vi "ROI entry-Event handler-Completion.vi"(7 "Adj Timing for MC":bool, 11 "Ctrl ref of the control that caused the user event":refnum<vi>) -> (1 "Exit":bool=TRUE, 3 "Imaging Mode":T1)   [LabVIEW 2020]
uses:
  Typedefs/Top level VI states.ctl
  Typedefs/Save-Load enum.ctl
  Typedefs/Which path.ctl
  Visualisation/Functional Imaging Viewer/SubVIs/Experiment header interface/Typedefs/Header file interface module functions enum.ctl
  Visualisation/Functional Imaging Viewer/SubVIs/Experiment header interface/Typedefs/Header file sections.ctl
  Visualisation/Functional Imaging Viewer/SubVIs/Experiment header interface/Typedefs/Header file type enum.ctl
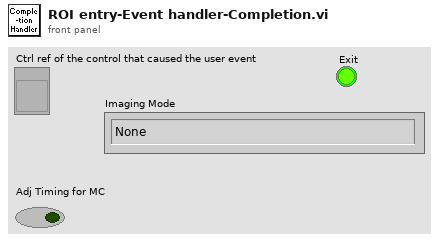
[diagram p1: front panel]
types:
  T1 = typedef "Top level VI states.ctl" = enum16{"None", "Initialise UI", "<STACK PROTOCOL STATES>", "AOL Zstack-START", "AOL Zstack-STOP", "Motor Zstack-START", "Motor Zstack-STOP", "<ACQUISITION PROTOCOL STATES> ", "Functional Acquisition-START", "Functional Acquisition-STOP", "Single Plane Acquisition-START", "Single Plane Acquisition-STOP", "Volume Acquisition-START", "Volume Acquisition-STOP", "<LIVE IMAGING PROTOCOL STATES>", "Live Imaging-START", "Live Imaging-STOP", "Live Plane Imaging-START", "Live Plane Imaging-STOP", "Live Volume Imaging-START", "Live Volume Imaging-STOP", "<MOVEMENT CORRECTION PROTOCOL STATES>", "EXIT"}
  T2 = typedef "Which path.ctl" = enum16{"Configuration Files", "Calibration Files", "Images", "Setup.ini", "Loaded User profile.ini", "User's-Previous session.ini", "New user profile.ini", "Selected User profile.ini", "User profiles folder", "Power meter scaling.txt", "FOV Cal.ini", "Calibration.ini"}
  T3 = typedef "Save-Load enum.ctl" = enum16{"Save to file", "Load from file", "Compare from file", "Save Backup"}
  T4 = typedef "Header file sections.ctl" = enum16{"ALL SECTIONS", "LOGIN", "GLOBAL PARAMETERS", "CALIBRATION DATA", "IMAGING MODES", "TIME SERIES", "MOTOR Z-STACK", "AOL Z-STACK", "FUNCTIONAL IMAGING", "VOLUME IMAGING", "MOVEMENT CORRECTION", "CALIBRATION", "STATISTICS", "BIOLOGY INFORMATION"}
  T5 = typedef "Header file interface module functions enum.ctl" = enum16{"Load experiment header file", "Save experiment header file", "Clear stored values", "Read stored values", "Update specific value in memory", "Update values in memory"}
  T6 = typedef "Header file type enum.ctl" = enum16{"All parameters", "Params for funct acq w ROI or mscn", "Params for funct acq w rectangles", "Live imaging header parameters", "AOL Parameters"}
  T7 = typedef "ROI parameters data type.ctl" = cluster{"ROI index":dbl, "ROI ID":dbl, "ROI Time (ns)":dbl, "Pixels in ROI":dbl, "X start":dbl, "Y start":dbl, "Z start":dbl, "X stop":dbl, "Y stop":dbl, "Z stop":dbl, "Angle (deg)":dbl, "Composite ID":dbl, "Number of lines":dbl, "Frame Size":dbl, "Zoom":dbl, "Laser Power (%)":dbl, "ROI group ID":dbl, "Resolution":dbl, "Dwell Time per pixel":dbl, "Pixels per miniscan":dbl, "Original FOV (um)":dbl, "Apparent Frame Size":dbl, "Z Plane Idx":i32[], "Z Plane codes":i32[]}
  T8 = typedef "AOL_Globals.ctl" = cluster{"Imaging Protocol":T9, "Number of POI":u16, "Number of Miniscans":u16, "Number of Trials":u16, "Number of Cycles ":u64, "# Averaged Frames":u16, "Laser power (%)":u8, "Pockels (V)":dbl, "Acquisition Length (sec)":dbl, "Fill time (us)":dbl, "POI Dwell time (us)":dbl, "Miniscan Dwell time per pixel (us)":dbl, "PMT 1":dbl, "PMT 2":dbl, "Back Apperture (mA)":dbl, "Frame Size":T10, "Center Frequency":dbl, "Field of View (norm)":dbl, "DwellTime (us)":dbl, "Wavelength (nm)":dbl, "Zoom":dbl, "AOL Z":dbl, "AOL Mode":T11, "GridXY":dbl, "GridZ":dbl, "TriggerPeriod (sec)":dbl, "Number of Pixels in Miniscan":u16, "Experiment folder path":path, "X centre":dbl, "Y centre":dbl, "Angle (degrees)":dbl, "Plane Mode":T12, "Threshold":u16[], "Regenerate Chirps":bool, "Rectangle ROI length (pixels)":u16, "Rectangle ROI height (pixels)":u16, "AOD fill":u16, "StartupDelay":i32, "Samples Wait after Trigger":u16, "Slip Cycle":u32, "Add Cycle":bool, "Functional Mode":T13, "Z Start":dbl, "Z Stop":dbl, "# Planes":i32, "Total Pixels":i32, "Variable Miniscan Pixels":u16[], "Use Variable Length":bool, "Use Variable Resolution":bool, "Laser power (%) at Z Start":u8, "Laser power (%) at Z Stop":u8, "Ref Z Step":i8, "Ref Dwell Time (us)":dbl, "Field of View (um)":dbl}
  T9 = typedef "Imaging Protocols enum.ctl" = enum16{"AOL Z-Stack", "Motor Z Stack", "Functional Acquisition", "Single Plane Acquisition", "Volume Acquisition", "Live Imaging", "Live Plane Imaging", "Live Volume Imaging"}
  T10 = typedef "Frame Size.ctl" = u16
  T11 = typedef "AOL modes.ctl" = enum16{"Raster", "Structural", "Pointing", "Mini Scan", "Alignment"}
  T12 = typedef "Plane Mode.ctl" = u16
  T13 = typedef "Functional Mode.ctl" = enum16{"Point", "Line", "Patch", "Plane", "Volume"}
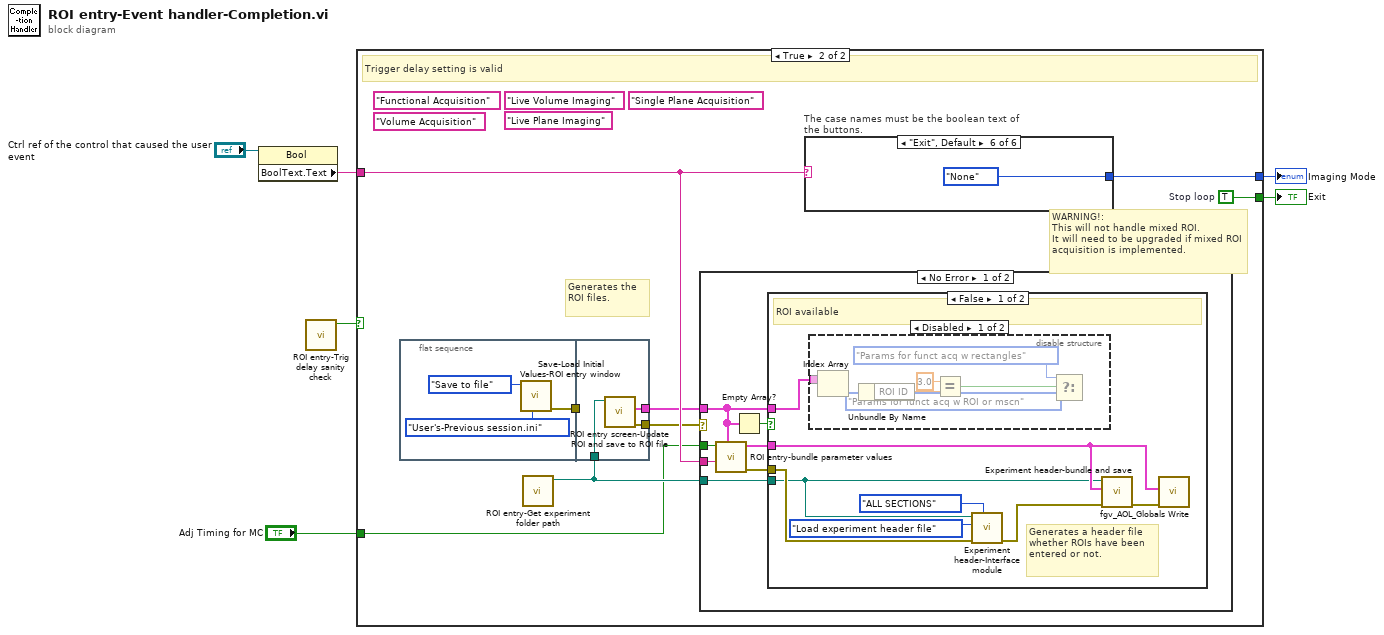
[diagram p0: block diagram]
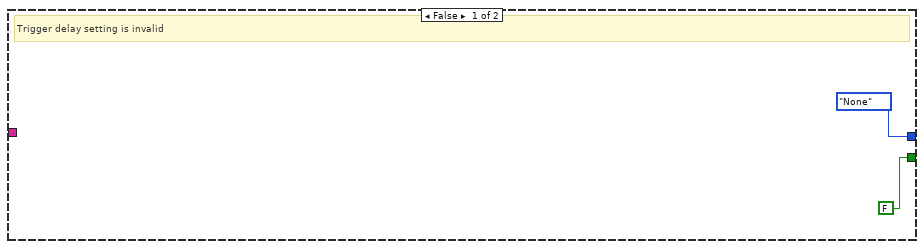
[diagram p2: hidden frame]
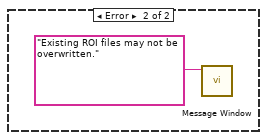
[diagram p5: hidden frame]
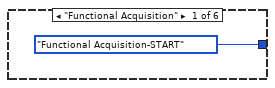
[diagram p6: hidden frame]
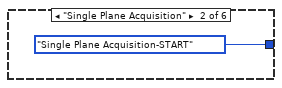
[diagram p7: hidden frame]
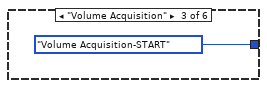
[diagram p8: hidden frame]
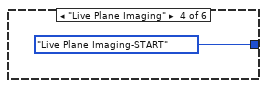
[diagram p9: hidden frame]
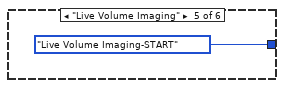
[diagram p10: hidden frame]
diagram:
  n1 = property on="Property Node" class="Bool"(reference="Ctrl ref of the control that caused the user event") -> ("BoolText.Text"=w6:string)  [unwired: 1 in, 2 out]
  n2 = call "ROI entry-Trig delay sanity check.vi"() -> ("Trigger delay is valid"=w2:bool)  [unwired: 10 in, 1 out]
  n3 = case shown="True" w2 {
    tunnel: w6 -> [_ w15]
    tunnel: [Top_level_VI_states."None" ("Imaging Mode") w12] -> w5
    tunnel: [FALSE ("Stop loop") w11] -> w3
    tunnel: "Adj Timing for MC" -> [_ w9]
    frame False {
      # "Trigger delay setting is invalid"
    }
    frame True {
      w11 = TRUE  # Stop loop
      (unwired) "Live Plane Imaging" ("Boolean Text.Text")
      (unwired) "Single Plane Acquisition" ("Boolean Text.Text")
      (unwired) "Live Volume Imaging" ("Boolean Text.Text")
      (unwired) "Functional Acquisition" ("Boolean Text.Text")
      (unwired) "Volume Acquisition" ("Boolean Text.Text")
      # "WARNING!:\nThis will not handle mixed ROI.\nIt will need to be upgraded if mixed ROI acquisition is implemented."
      # "Generates the ROI files."
      # "Trigger delay setting is valid"
      n4 = flat-sequence {
        tunnel: [w17] -> w10
        tunnel: w16 -> [w22]
        tunnel: [w21] -> w14
        tunnel: [w20] -> w13
        tunnel: w10 -> [_]
        frame #0 {
          n5 = call "Save-Load Initial Values-ROI entry window.vi"("Which file? (User profile.ini)"=Which_path."User's-Previous session.ini", "Function"=Save-Load_enum."Save to file") -> ("error out"=w17:errorcluster)  [unwired: 9 in]
        }
        frame #1 {
          n6 = call "ROI entry screen-Update ROI and save to ROI file.vi"("Experiment folder path"=w22) -> ("Error Out"=w21:errorcluster, "XYZ_Coordinates"=w20:T7[])  [unwired: 9 in]
        }
      }
      n7 = call "ROI entry-Get experiment folder path.vi"() -> ("Experiment folder path"=w16:path)  [unwired: 10 in, 1 out]
      n8 = case shown="No Error" w14 {
        tunnel: w13 -> [w24 _]
        tunnel: w16 -> [w29 _]
        tunnel: w15 -> [w25 _]
        tunnel: w9 -> [w23 _]
        frame No Error {
          n9 = call "ROI entry-bundle parameter values.vi"("XYZ_Coordinates"=w24, "Button Label.Text"=w25, "Adj Timing for MC"=w23) -> ("error out"=w27:errorcluster, "AOL_Globals out"=w28:T8)  [unwired: 7 in]
          n10 = Empty Array?(array=w24) -> (empty?=w26:bool)
          n11 = case shown="False" w26 {
            tunnel: w29 -> [w31 _]
            tunnel: w28 -> [w36 _]
            tunnel: w27 -> [w32 _]
            tunnel: w24 -> [w35 _]
            frame False {
              # "Generates a header file whether ROIs have been entered or not."
              # "ROI available"
              n12 = disable-structure shown="Disabled" {
                disable-tunnel: w35 -> [w44 _]
                frame Disabled {
                  n13 = Index Array(array=w44) -> (element=w43:T7)  [unwired: 1 in]
                  n14 = Unbundle By Name(w43) -> ("ROI ID"=w42:dbl)
                  n15 = Equal?(x=3.0 ("y"), y=w42) -> (x = y?=w40:bool)
                  n16 = Select(t=Header_file_type_enum."Params for funct acq w rectangles" ("Header file type"), s=w40, f=Header_file_type_enum."Params for funct acq w ROI or mscn" ("Header file type")) -> ()  [unwired: 1 out]
                }
                frame Enabled {
                }
              }
              n17 = call "Experiment header-Interface module.vi"("Header file sections"=Header_file_sections."ALL SECTIONS", "error in (no error)"=w32, "Function"=Header_file_interface_module_functions_enum."Load experiment header file", "Experiment data folder path"=w31) -> ("error out"=w30:errorcluster)  [unwired: 6 in, 1 out]
              n18 = call "Experiment header-bundle and save.vi"("error in (no error)"=w30, "AOL_Globals"=w36, "Experiment data folder path"=w31) -> ("error out"=w37:errorcluster)  [unwired: 8 in]
              n19 = call "fgv_AOL_Globals Write.vi"("error in (no error)"=w37, "AOL_Globals"=w36) -> ()  [unwired: 9 in, 1 out]
            }
            frame True {
              # "NO ROI ENTERED"
            }
          }
        }
        frame Error {
          n20 = call "Message Window.vi"("Message string"="Existing ROI files may not be overwritten.") -> ()  [unwired: 10 in, 1 out]
        }
      }
      n21 = case "The case names must be the boolean text of the buttons." shown="\"Exit\", Default" w15 {
        tunnel: [Top_level_VI_states."Functional Acquisition-START" ("Imaging Mode") Top_level_VI_states."Single Plane Acquisition-START" ("Imaging Mode") Top_level_VI_states."Volume Acquisition-START" ("Imaging Mode") Top_level_VI_states."Live Plane Imaging-START" ("Imaging Mode") Top_level_VI_states."Live Volume Imaging-START" ("Imaging Mode") Top_level_VI_states."None" ("Imaging Mode")] -> w12
        frame "Functional Acquisition" {
        }
        frame "Single Plane Acquisition" {
        }
        frame "Volume Acquisition" {
        }
        frame "Live Plane Imaging" {
        }
        frame "Live Volume Imaging" {
        }
        frame "Exit", Default {
        }
      }
    }
  }
  "Imaging Mode" <- w5
  "Exit" <- w3
